vi "Defer Updates.vi"(8 "Error In":errorcluster, 11 "Panel Actor in":refnum<class "Panel Actor.lvclass">) -> (0 "Error Out":errorcluster, 2 "Deferer":refnum<class "Deferer.lvclass">)   [LabVIEW 2017, in "MGI-Panel Actor.lvlib" / "Panel Actor.lvclass"]
doc: "Defers updates for the panel.\n\n<B>Controller In:</B> Panel Helper object to handle Defer\n<B>Error In:</B> Describes error conditions that occur before this node runs.\n\n<B>Deferer:</B> Deferer object.\n<B>Error Out:</B> Contains error information.\n----\nCopyright: MGI 2018\nAuthor: Derek Trepanier"
uses:
  Panel Actor.lvclass
  panel-manager/Source/Panel Helper/Panel Helper.lvclass
  panel-manager/Source/Deferer/Deferer.lvclass
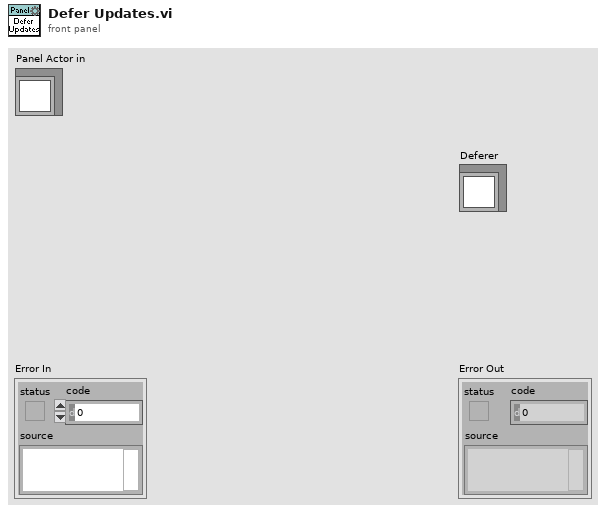
[diagram p1: front panel]
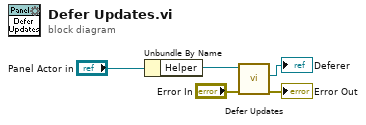
[diagram p0: block diagram]
diagram:
  n1 = Unbundle By Name("Panel Actor in") -> ("Helper"=w4:refnum<class "Panel Helper.lvclass">)
  n2 = call "Defer Updates.vi"("Error In"="Error In", "Controller in"=w4) -> ("Error Out"=→"Error Out":errorcluster, "Deferer"=→"Deferer":refnum<class "Deferer.lvclass">)  [unwired: 8 in]
